vi "Start Test Selection (SubVI).vi"(8 "error in (no error)":errorcluster, 9 "TestArrayIn":string[](array[string])) -> (1 "AutoOut":bool, 2 "TestArrayOut":string[](array[string]))   [LabVIEW 2017]
panel:
  in  "Next Button":bool
  in  "Auto":bool
  in  "Listbox":i32[](listbox)
  # "Use Ctrl key to select many."
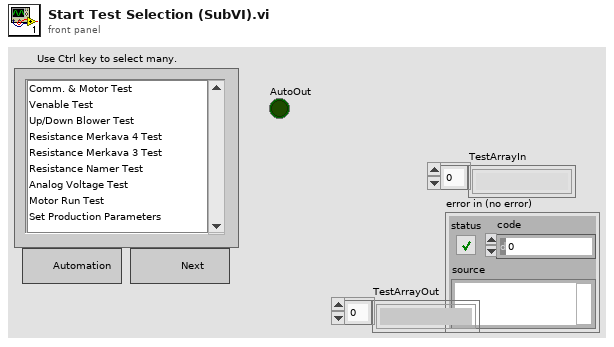
[diagram p1: front panel]
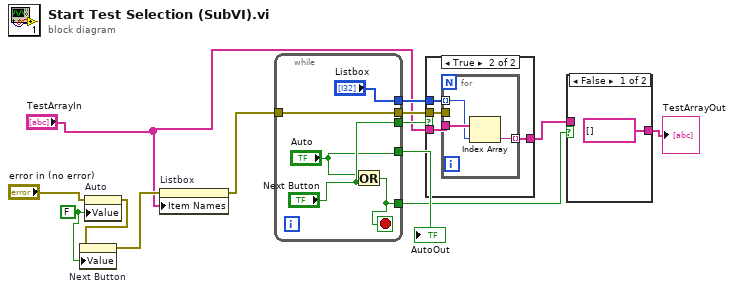
[diagram p0: block diagram]
diagram:
  w10 = FALSE ("Auto")
  n1 = property on="Auto" class="Bool (strict)"(error in="error in (no error)", "Value"=w10) -> (error out=w8:errorcluster)  [unwired: 1 in, 1 out]
  n2 = property on="Next Button" class="Bool (strict)"(error in=w8, "Value"=w10) -> (error out=w7:errorcluster)  [unwired: 1 in, 1 out]
  n3 = property on="Listbox" class="LstBox (strict)"(error in=w7, "Item Names"="TestArrayIn") -> (error out=w12:errorcluster)  [unwired: 1 in, 1 out]
  n4 = while {
    tunnel: ["Listbox"] -> w13
    tunnel: w12 -> [w17]
    tunnel: [w17] -> w11
    tunnel: ["Next Button"] -> w6
    tunnel: ["Auto"] -> w5
    tunnel: [w14] -> w3
    stop <- w14 stop-if-true
    n5 = Or(x="Auto", y="Next Button") -> (x .or. y?=w14:bool)
  }
  "AutoOut" <- w5
  n6 = case shown="True" w6 {
    tunnel: w13 -> [_ w23]
    tunnel: "TestArrayIn" -> [w19 w22]
    tunnel: w11 -> [_ w21]
    tunnel: [w19 w20] -> w2
    frame False {
    }
    frame True {
      n7 = for {
        tunnel: w23 -> [w24] mode=indexing
        tunnel: [w25] -> w20 mode=indexing
        tunnel: w22 -> [w26]
        tunnel: w21 -> [_]
        n8 = Index Array(array=w26, index=w24) -> (element=w25:string)
      }
    }
  }
  n9 = case shown="False" w3 {
    tunnel: [string[] [] ("TestArrayIn") w28] -> w1
    tunnel: w2 -> [_ w28]
    frame False {
    }
    frame True {
    }
  }
  "TestArrayOut" <- w1
